vi "optimise_motor_position.vi"(0 "address":string, 1 "Crystal Speed / counts s-1":dbl, 5 "Crystal Number":u16(ring) items=["Crystal 1", "Crystal 2", "Crystal 3", "Crystal 4", "Crystal 5", "Crystal 6", "Crystal 7", ""], 7 "Start Position":i32, 9 "End Position":i32, 11 "error in":errorcluster) -> (6 "Crystal Number Out":i32, 8 "Opimised Position":i32)   [LabVIEW 2020]
panel:
  out "error out":errorcluster
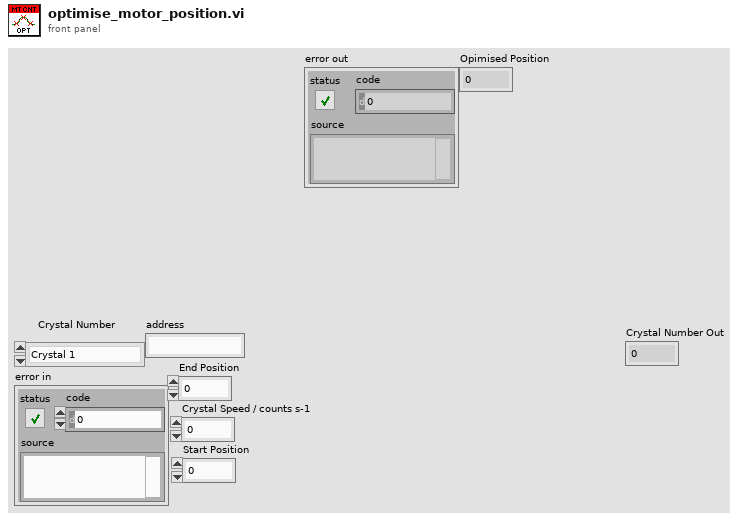
[diagram p1: front panel]
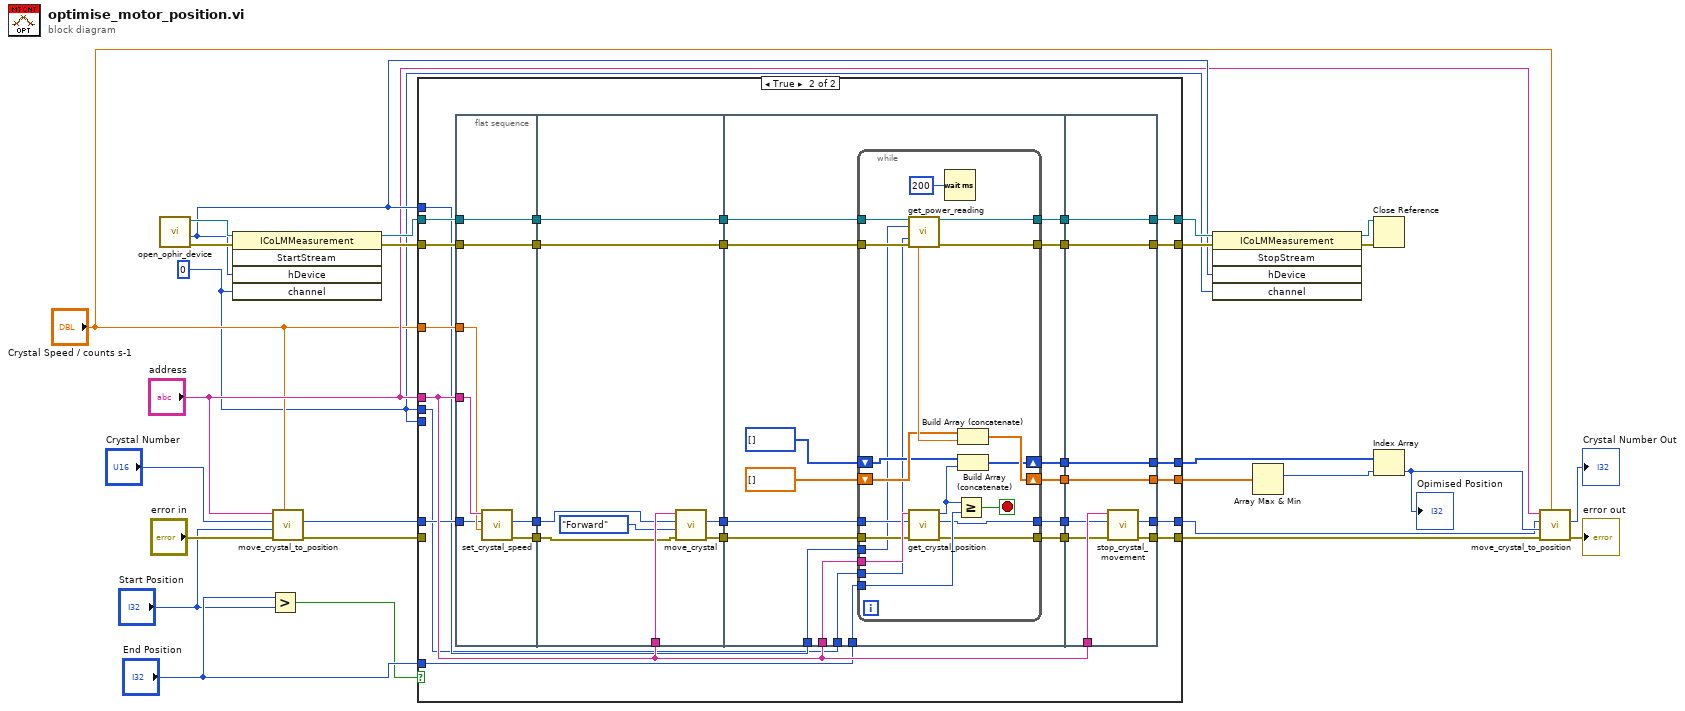
[diagram p0: block diagram]
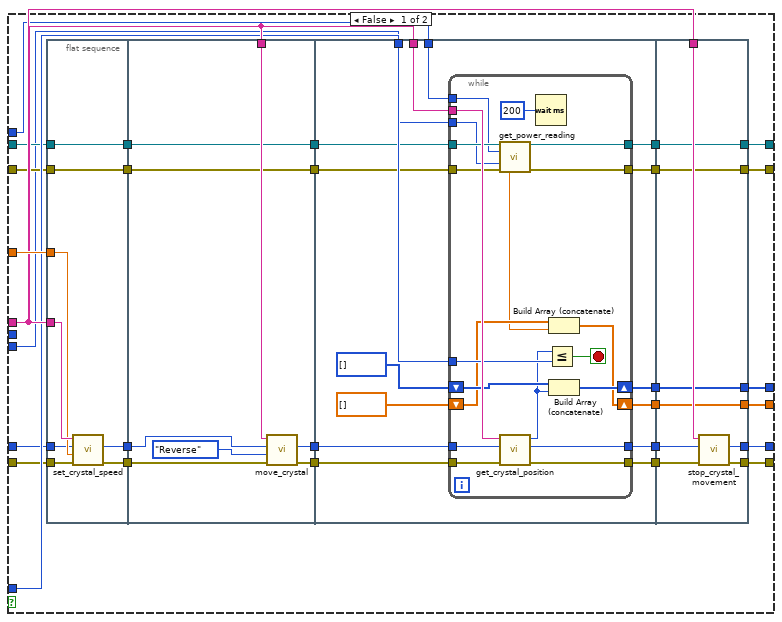
[diagram p2: hidden frame]
diagram:
  w1 = 0 ("channel")
  n1 = call "open_ophir_device.vi"() -> ("error out"=w20:errorcluster, "hDevice"=w13:i32, "Orphir COM"=w21:refnum<k7>)  [unwired: 7 in, 2 out]
  n2 = invoke class="ICoLMMeasurement" method="StartStream"(reference=w21, error in=w20, "hDevice"=w13, "channel"=w1) -> (reference out=w19:refnum<k7>, error out=w18:errorcluster)  [unwired: 1 in, 3 out]
  n3 = Greater?(x="End Position", y="Start Position") -> (0:w26:bool)
  n4 = call "move_crystal_to_position.vi"("Crystal Speed / counts s-1"="Crystal Speed / counts s-1", "error in"="error in", "Desired Position"="Start Position", "Crystal Number"="Crystal Number", "address"="address") -> ("error out"=w22:errorcluster, "Crystal Number Out"=w23:i32)  [unwired: 5 in]
  n5 = case shown="True" w26 {
    tunnel: "address" -> [w48 w140]
    tunnel: "Crystal Speed / counts s-1" -> [w49 w141]
    tunnel: [w50 w137] -> w6
    tunnel: [w51 w136] -> w3
    tunnel: "End Position" -> [w47 w135]
    tunnel: w23 -> [w45 w120]
    tunnel: w22 -> [w44 _]
    tunnel: w19 -> [w43 w132]
    tunnel: w18 -> [w38 w129]
    tunnel: [w36 w122] -> w15
    tunnel: [w34 w121] -> w14
    tunnel: w13 -> [w33 w119]
    tunnel: w1 -> [w32 _]
    tunnel: [w29 w124] -> w11
    tunnel: [w28 w123] -> w12
    tunnel: w1 -> [_ w118]
    frame False {
      n6 = flat-sequence {
        tunnel: w48 -> [w64]
        tunnel: [w63] -> w56
        tunnel: [w62] -> w55
        tunnel: w49 -> [w61]
        tunnel: w45 -> [w60]
        tunnel: w44 -> [w59]
        tunnel: w43 -> [w58]
        tunnel: [w58] -> w41
        tunnel: [w57] -> w39
        tunnel: w38 -> [w57]
        tunnel: w48 -> [w72]
        tunnel: w56 -> [w71]
        tunnel: [w70] -> w54
        tunnel: w55 -> [w69]
        tunnel: [w68] -> w53
        tunnel: [w66] -> w42
        tunnel: w41 -> [w66]
        tunnel: [w65] -> w40
        tunnel: w39 -> [w65]
        tunnel: w48 -> [w88]
        tunnel: w54 -> [w87]
        tunnel: w53 -> [w86]
        tunnel: [w85] -> w52
        tunnel: w47 -> [w84]
        tunnel: [w83] -> w46
        tunnel: w42 -> [w81]
        tunnel: w40 -> [w80]
        tunnel: [w79] -> w37
        tunnel: [w78] -> w35
        tunnel: w33 -> [w77]
        tunnel: w32 -> [w76]
        tunnel: [w74] -> w31
        tunnel: [w73] -> w30
        tunnel: w48 -> [w117]
        tunnel: w52 -> [w116]
        tunnel: [w115] -> w50
        tunnel: [w114] -> w51
        tunnel: w46 -> [w113]
        tunnel: w37 -> [w112]
        tunnel: [w112] -> w36
        tunnel: [w111] -> w34
        tunnel: w35 -> [w111]
        tunnel: w31 -> [w110]
        tunnel: [w110] -> w29
        tunnel: w30 -> [w109]
        tunnel: [w109] -> w28
        frame #0 {
          n7 = call "set_crystal_speed.vi"("error in"=w59, "Crystal Speed / counts s-1"=w61, "Crystal Number"=w60, "address"=w64) -> ("error out"=w62:errorcluster, "Crystal Number Out"=w63:u16)  [unwired: 6 in]
        }
        frame #1 {
          n8 = call "move_crystal.vi"("error in"=w69, "Direction"=enum16{"Reverse", "Forward"}."Reverse", "Crystal Number"=w71, "address"=w72) -> ("error out"=w70:errorcluster, "Crystal Number Out"=w68:u16)  [unwired: 6 in]
        }
        frame #2 {
          n9 = while {
            tunnel: w88 -> [w108]
            tunnel: w87 -> [w107]
            tunnel: w86 -> [w106]
            tunnel: [w103] -> w85
            tunnel: w84 -> [w102]
            tunnel: [w101] -> w83
            shift-right: [w99] -> w74
            shift-left: i32[] [] -> [w100]
            tunnel: w81 -> [w97]
            tunnel: w80 -> [w96]
            tunnel: [w95] -> w79
            tunnel: [w94] -> w78
            tunnel: w77 -> [w93]
            tunnel: w76 -> [w92]
            shift-right: [w90] -> w73
            shift-left: dbl[] [] -> [w91]
            stop <- w104 stop-if-true
            n10 = call "get_power_reading.vi"("reference in"=w97, "hDevice"=w93, "channel"=w92, "error in (no error)"=w96) -> ("reference out"=w95:refnum<k7>, "Power / J"=w89:dbl, "error out"=w94:errorcluster)  [unwired: 5 in, 4 out]
            n11 = call "get_crystal_position.vi"("error in"=w107, "Crystal Number"=w106, "address"=w108) -> ("error out"=w103:errorcluster, "Crystal Number Out"=w101:u16, "Crystal Position"=w98:i32)  [unwired: 6 in]
            n12 = Wait (ms)(milliseconds to wait=u32 200) -> ()  [unwired: 1 out]
            n13 = Less Or Equal?(x=w98, y=w102) -> (x <= y?=w104:bool)
            n14 = Build Array (concatenate)(w91, w89) -> (w90:dbl[])
            n15 = Build Array (concatenate)(w100, w98) -> (w99:i32[])
          }
        }
        frame #3 {
          n16 = call "stop_crystal_movement.vi"("error in"=w116, "Crystal Number"=w113, "address"=w117) -> ("error out"=w115:errorcluster, "Crystal Number Out"=w114:u16)  [unwired: 7 in]
        }
      }
    }
    frame True {
      n17 = flat-sequence {
        tunnel: w140 -> [w152]
        tunnel: [w151] -> w145
        tunnel: [w150] -> w143
        tunnel: w141 -> [w149]
        tunnel: [w148] -> w133
        tunnel: w132 -> [w148]
        tunnel: w129 -> [w147]
        tunnel: [w147] -> w131
        tunnel: w120 -> [w146]
        tunnel: w140 -> [w160]
        tunnel: w145 -> [w159]
        tunnel: [w158] -> w144
        tunnel: w143 -> [w157]
        tunnel: [w156] -> w142
        tunnel: [w154] -> w134
        tunnel: w133 -> [w154]
        tunnel: w131 -> [w153]
        tunnel: [w153] -> w130
        tunnel: w140 -> [w176]
        tunnel: w144 -> [w175]
        tunnel: w142 -> [w174]
        tunnel: w135 -> [w173]
        tunnel: [w172] -> w139
        tunnel: [w171] -> w138
        tunnel: w134 -> [w170]
        tunnel: w130 -> [w169]
        tunnel: [w168] -> w128
        tunnel: [w167] -> w127
        tunnel: [w164] -> w126
        tunnel: [w163] -> w125
        tunnel: w119 -> [w162]
        tunnel: w118 -> [w161]
        tunnel: w140 -> [w205]
        tunnel: w139 -> [w204]
        tunnel: w138 -> [w203]
        tunnel: [w202] -> w137
        tunnel: [w201] -> w136
        tunnel: [w200] -> w122
        tunnel: w128 -> [w200]
        tunnel: [w199] -> w121
        tunnel: w127 -> [w199]
        tunnel: [w198] -> w124
        tunnel: w126 -> [w198]
        tunnel: [w197] -> w123
        tunnel: w125 -> [w197]
        frame #0 {
          n18 = call "set_crystal_speed.vi"("Crystal Speed / counts s-1"=w149, "Crystal Number"=w146, "address"=w152) -> ("error out"=w150:errorcluster, "Crystal Number Out"=w151:u16)  [unwired: 7 in]
        }
        frame #1 {
          n19 = call "move_crystal.vi"("error in"=w157, "Direction"=enum16{"Reverse", "Forward"}."Forward", "Crystal Number"=w159, "address"=w160) -> ("error out"=w158:errorcluster, "Crystal Number Out"=w156:u16)  [unwired: 6 in]
        }
        frame #2 {
          n20 = while {
            tunnel: w176 -> [w196]
            tunnel: w175 -> [w195]
            tunnel: w174 -> [w194]
            tunnel: w173 -> [w192]
            tunnel: [w190] -> w172
            tunnel: [w189] -> w171
            tunnel: w170 -> [w188]
            tunnel: w169 -> [w187]
            tunnel: [w186] -> w168
            tunnel: [w185] -> w167
            shift-right: [w182] -> w163
            shift-left: dbl[] [] -> [w183]
            shift-right: [w180] -> w164
            shift-left: i32[] [] -> [w181]
            tunnel: w162 -> [w178]
            tunnel: w161 -> [w177]
            stop <- w191 stop-if-true
            n21 = call "get_power_reading.vi"("reference in"=w188, "hDevice"=w178, "channel"=w177, "error in (no error)"=w187) -> ("reference out"=w186:refnum<k7>, "Power / J"=w184:dbl, "error out"=w185:errorcluster)  [unwired: 5 in, 4 out]
            n22 = call "get_crystal_position.vi"("error in"=w195, "Crystal Number"=w194, "address"=w196) -> ("error out"=w189:errorcluster, "Crystal Number Out"=w190:u16, "Crystal Position"=w179:i32)  [unwired: 6 in]
            n23 = Wait (ms)(milliseconds to wait=u32 200) -> ()  [unwired: 1 out]
            n24 = Greater Or Equal?(x=w179, y=w192) -> (x >= y?=w191:bool)
            n25 = Build Array (concatenate)(w183, w184) -> (w182:dbl[])
            n26 = Build Array (concatenate)(w181, w179) -> (w180:i32[])
          }
        }
        frame #3 {
          n27 = call "stop_crystal_movement.vi"("error in"=w203, "Crystal Number"=w204, "address"=w205) -> ("error out"=w202:errorcluster, "Crystal Number Out"=w201:u16)  [unwired: 7 in]
        }
      }
    }
  }
  n28 = invoke class="ICoLMMeasurement" method="StopStream"(reference=w15, error in=w14, "hDevice"=w13, "channel"=w1) -> (reference out=w17:refnum<k7>, error out=w16:errorcluster)  [unwired: 1 in, 3 out]
  n29 = Array Max & Min(array=w12) -> (max index (indices)=w10:i32)  [unwired: 3 out]
  n30 = Close Reference(reference=w17, error in (no error)=w16) -> ()  [unwired: 1 out]
  n31 = Index Array(array=w11, index=w10) -> (element=w9:i32)
  "Opimised Position" <- w9
  n32 = call "move_crystal_to_position.vi"("Crystal Speed / counts s-1"="Crystal Speed / counts s-1", "error in"=w6, "Desired Position"=w9, "Crystal Number"=w3, "address"="address") -> ("error out"=→"error out":errorcluster, "Crystal Number Out"=→"Crystal Number Out":i32)  [unwired: 5 in]
